vi "CheckData.vi"(9 "upper limit":dbl=1.0 format="%#_13g", 10 "lower limit":dbl=-1.0 format="%#_13g", 11 "read buffer":string) -> (2 "number":dbl, 3 "Boolean":bool)   [LabVIEW 2017]
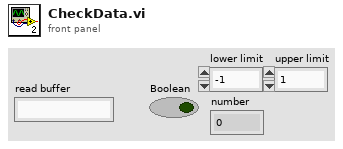
[diagram p1: front panel]
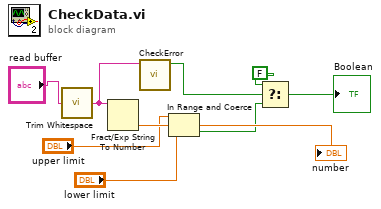
[diagram p0: block diagram]
diagram:
  n1 = call <vilib>:"Trim Whitespace.vi"("string"="read buffer") -> ("trimmed string"=w5:string)  [unwired: 1 in]
  n2 = Fract/Exp String To Number(string=w5) -> (number=w9:dbl)  [unwired: 3 in, 1 out]
  "number" <- w9
  n3 = call "CheckError.vi"("Data string"=w5) -> ("T Error"=w4:bool)  [unwired: 10 in]
  n4 = In Range and Coerce(upper limit="upper limit", x=w9, lower limit="lower limit") -> (In Range?=w2:bool)  [unwired: 1 out]
  n5 = Select(t=FALSE, s=w4, f=w2) -> (s? t:f=→"Boolean":bool)
